vi "2.1.vi"() -> ()   [LabVIEW 2017]
uses:
  <vilib>/express/express shared/transition.llb/Dynamic To Waveform Array.vi
  <vilib>/express/express arith-compare/Formula/Block/exnFormulaBlock how many pts in the wave.vi
  <vilib>/express/express shared/ex_Modify Signal Name.vi
  <vilib>/express/express shared/transition.llb/Waveform Array To Dynamic.vi
  <vilib>/express/express arith-compare/Formula/XNode/ExpressFormulaBlockNode.xnode
panel:
  in  "stop":bool
  out "Waveform Chart":dynamicdata(graph)
  in  "X3":dbl
  in  "X2":dbl
  in  "Амплитуда":dbl(knob) scale=0.0..10.0
  in  "Частота":dbl(knob) scale=0.0..10.0
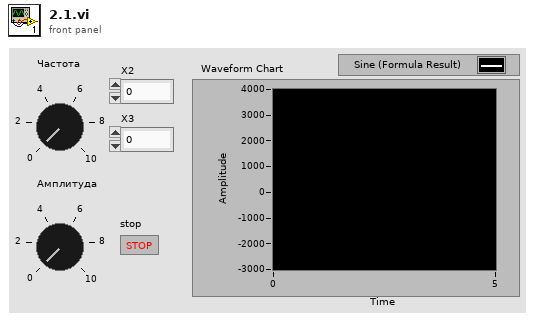
[diagram p1: front panel]
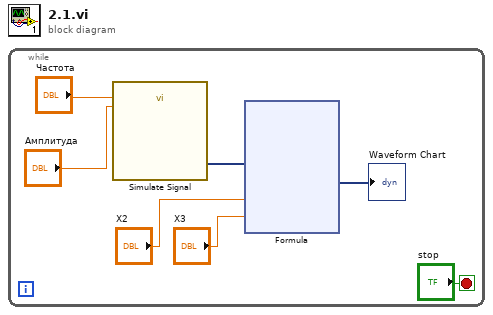
[diagram p0: block diagram]
diagram:
  n1 = while {
    stop <- "stop" stop-if-true
    n2 = call "Simulate Signal"("Frequency"="Частота", "Amplitude"="Амплитуда") -> ("Sine"=w2:dynamicdata)  [unwired: 12 in, 1 out]
    n3 = xnode "Formula"("X1"=w2, "X2"="X2", "X3"="X3") -> ("Result"=→"Waveform Chart":dynamicdata)  [unwired: 1 in, 1 out]
  }
